vi "Keithley_test_JPV.vi"(2 "Function (0: DC Volts)":u16, 3 "VISA resource name":refnum<visa-resource-name>) -> (0 "error out":errorcluster, 1 "Measurement":dbl)   [LabVIEW 2018]
uses:
  Public/Configure/Configure DC Volts.vi
  Public/Configure/Configure AC Volts.vi
  Public/Configure/Configure DC Current.vi
  Public/Configure/Configure AC Current.vi
  Public/Configure/Configure 2 Wire Resistance.vi
  Public/Configure/Configure 4 Wire Resistance.vi
  Keithley 2100 Series.lvlib
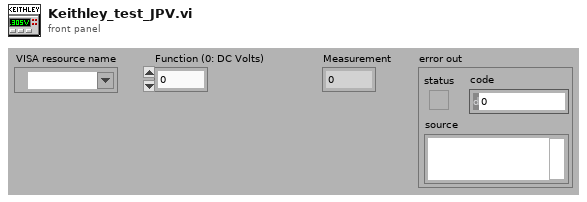
[diagram p1: front panel]
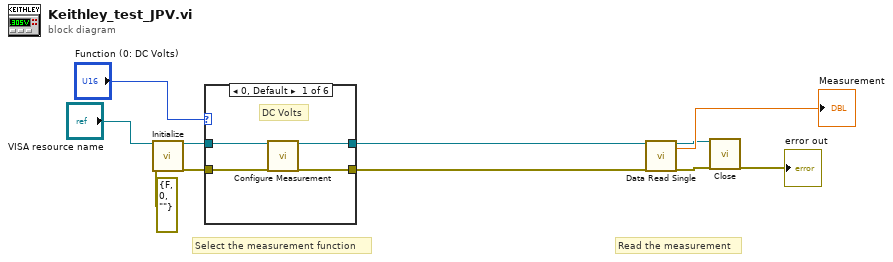
[diagram p0: block diagram]
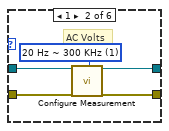
[diagram p2: hidden frame]
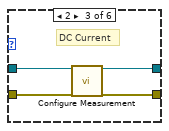
[diagram p3: hidden frame]
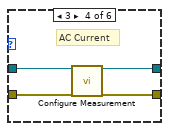
[diagram p4: hidden frame]
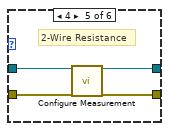
[diagram p5: hidden frame]
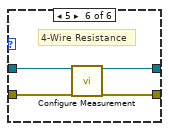
[diagram p6: hidden frame]
diagram:
  # "Read the measurement"
  # "Select the measurement function"
  n1 = call "Initialize.vi"("VISA resource name"="VISA resource name", "error in (no error)"=errorcluster {"status"=FALSE, "code"=0, "source"=""}) -> ("VISA resource name out"=w4:refnum<visa-resource-name>, "error out"=w1:errorcluster)  [unwired: 16 in]
  n2 = case shown="0, Default" "Function (0: DC Volts)" {
    tunnel: w1 -> [w15 w20 w24 w28 w32 w36]
    tunnel: w4 -> [w14 w19 w23 w27 w31 w35]
    tunnel: [w13 w18 w22 w26 w30 w34] -> w11
    tunnel: [w12 w17 w21 w25 w29 w33] -> w10
    frame 0, Default {
      # "DC Volts"
      n3 = call-poly "Configure Measurement.vi"("VISA resource name"=w14, "error in (no error)"=w15) -> ("VISA resource name out"=w12:refnum<visa-resource-name>, "error out"=w13:errorcluster)  [unwired: 16 in]
    }
    frame 1 {
      w16 = u16 1 items=["3 Hz ~ 300 KHz", "20 Hz ~ 300 KHz", "200 Hz ~ 300 KHz"] ("Bandwidth (20 Hz)")
      # "AC Volts"
      n4 = call-poly "Configure Measurement.vi"("VISA resource name"=w19, "error in (no error)"=w20, "Bandwidth (20 Hz)"=w16) -> ("VISA resource name out"=w17:refnum<visa-resource-name>, "error out"=w18:errorcluster)  [unwired: 15 in]
    }
    frame 2 {
      # "DC Current"
      n5 = call-poly "Configure Measurement.vi"("VISA resource name"=w23, "error in (no error)"=w24) -> ("VISA resource name out"=w21:refnum<visa-resource-name>, "error out"=w22:errorcluster)  [unwired: 16 in]
    }
    frame 3 {
      # "AC Current"
      n6 = call-poly "Configure Measurement.vi"("VISA resource name"=w27, "error in (no error)"=w28) -> ("VISA resource name out"=w25:refnum<visa-resource-name>, "error out"=w26:errorcluster)  [unwired: 16 in]
    }
    frame 4 {
      # "2-Wire Resistance"
      n7 = call-poly "Configure Measurement.vi"("VISA resource name"=w31, "error in (no error)"=w32) -> ("VISA resource name out"=w29:refnum<visa-resource-name>, "error out"=w30:errorcluster)  [unwired: 16 in]
    }
    frame 5 {
      # "4-Wire Resistance"
      n8 = call-poly "Configure Measurement.vi"("VISA resource name"=w35, "error in (no error)"=w36) -> ("VISA resource name out"=w33:refnum<visa-resource-name>, "error out"=w34:errorcluster)  [unwired: 16 in]
    }
  }
  n9 = call "Data Read Single.vi"("VISA resource name"=w10, "error in (no error)"=w11) -> ("VISA resource name out"=w3:refnum<visa-resource-name>, "Measurement"=→"Measurement":dbl, "error out"=w2:errorcluster)  [unwired: 15 in]
  n10 = call "Close.vi"("VISA resource name"=w3, "error in (no error)"=w2) -> ("error out"=→"error out":errorcluster)  [unwired: 17 in]
